vi "PH_Sound.Device Play Wave.vi"(3 "error in (no error)":errorcluster, 5 "path":path) -> (0 "Device error out":errorcluster)   [LabVIEW 2014, in "PH_Sound.lvlib"]
uses:
  PH_Sound.lvlib
  <vilib>/sound2/lvsound2.llb/Sampling Mode.ctl
  <vilib>/sound2/lvsound2.llb/Sound File Info (path).vi
  <vilib>/sound2/lvsound2.llb/Sound File Read Open.vi
  <vilib>/sound2/lvsound2.llb/Sound File Read (DBL).vi
  <vilib>/sound2/lvsound2.llb/Sound Output Write (DBL).vi
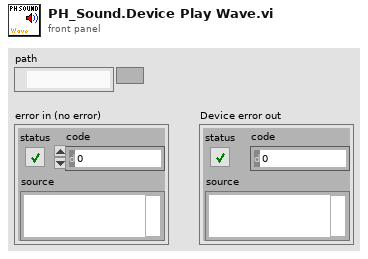
[diagram p1: front panel]
types:
  T1 = typedef "Sampling Mode.ctl" = i32
  T2 = typedef "Sound Data Format.ctl" = cluster{"sample rate (S/s)":dbl, "number of channels":i32, "bits per sample":i32}
  T3 = typedef "Sound File Refnum.ctl" = refnum<file>
  T4 = typedef "Sound Output Task ID.ctl" = u32
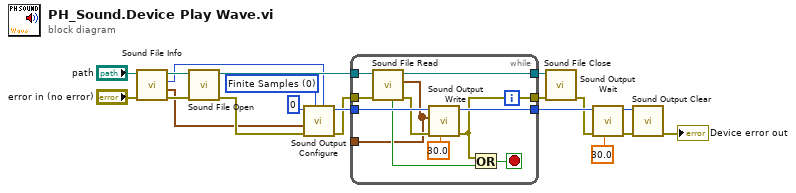
[diagram p0: block diagram]
diagram:
  w4 = T1 0 items=["Finite Samples", "Continuous Samples"] ("sample mode")
  n1 = call-poly <vilib>:"Sound File Info.vi"("error in (no error)"="error in (no error)", "path"="path") -> ("error out"=w9:errorcluster, "sound format"=w3:T2, "total number of samples/ch"=w1:u32, "path out"=w10:path)  [unwired: 6 in]
  n2 = call-poly <vilib>:"Sound File Open.vi"("error in (no error)"=w9, "path"=w10) -> ("error out"=w7:errorcluster, "sound file refnum"=w14:T3)  [unwired: 8 in]
  n3 = call <vilib>:"Sound Output Configure.vi"("number of samples/ch"=w1, "sample mode"=w4, "error in (no error)"=w7, "sound format"=w3, "device ID"=u32 0) -> ("error out"=w6:errorcluster, "task ID"=w8:T4)  [unwired: 5 in]
  n4 = while {
    tunnel: w14 -> [w29]
    tunnel: [w28] -> w16
    tunnel: w6 -> [w30]
    tunnel: [w23] -> w15
    tunnel: w8 -> [w27]
    tunnel: [w31] -> w13
    tunnel: [w21] -> _
    stop <- w24 stop-if-true
    # "Read Sound File and Generate Sound"
    n5 = call-poly <vilib>:"Sound File Read.vi"("error in (no error)"=w30, "sound file refnum"=w29) -> ("error out"=w26:errorcluster, "data"=w21:waveform(dbl)[], "sound file refnum out"=w28:T3, "end of file?"=w25:bool)  [unwired: 5 in, 1 out]
    n6 = call-poly <vilib>:"Sound Output Write.vi"("timeout (sec)"=30.0, "error in (no error)"=w26, "data"=w21, "task ID"=w27) -> ("error out"=w23:errorcluster, "task ID out"=w31:T4)  [unwired: 6 in]
    n7 = Or(x=w23, y=w25) -> (x .or. y?=w24:bool)
  }
  n8 = call <vilib>:"Sound File Close.vi"("error in (no error)"=w15, "sound file refnum"=w16) -> ("error out"=w12:errorcluster)  [unwired: 9 in]
  n9 = call <vilib>:"Sound Output Wait.vi"("timeout (sec)"=30.0, "error in (no error)"=w12, "task ID"=w13) -> ("error out"=w11:errorcluster, "task ID out"=w5:T4)  [unwired: 7 in]
  n10 = call <vilib>:"Sound Output Clear.vi"("error in (no error)"=w11, "task ID"=w5) -> ("error out"=→"Device error out":errorcluster)  [unwired: 9 in]
